vi "Add DataRow to Table by Values.vi"(8 "error in (no error)":errorcluster caption="错误输入（无错误）", 10 "values":variant[](array[variant]), 11 "DataTable 输入":refnum<class "DataTable.lvclass"> caption="DNL_LabVIEW Object in") -> (0 "error out":errorcluster caption="错误输出", 3 "DataTable 输出":refnum<class "DataTable.lvclass"> caption="DNL_LabVIEW Object out")   [LabVIEW 2012, in "Data Grid VIEW.lvlib" / "DataTable.lvclass"]
uses:
  DataTable.lvclass
  DataTable.lvclass/DataTable.ctl
  System.Data
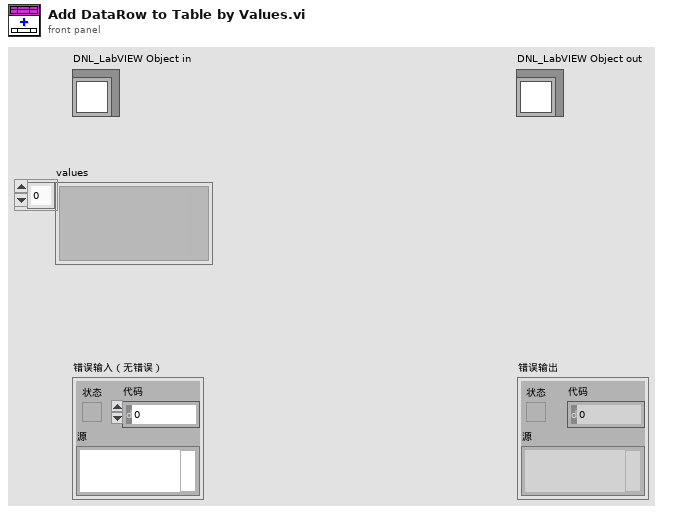
[diagram p1: front panel]
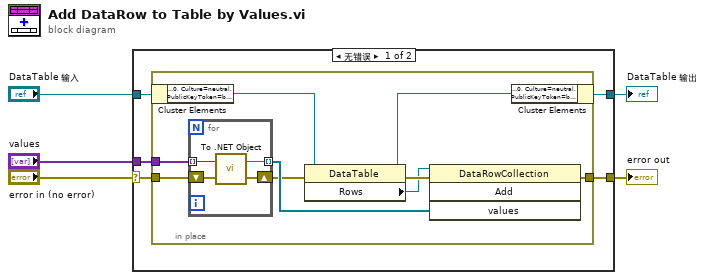
[diagram p0: block diagram]
diagram:
  n1 = case shown="无错误" "error in (no error)" {
    selector: "error in (no error)" -> [w8 w25]
    tunnel: [w7 w25] -> w4
    tunnel: [w6 w24] -> w2
    tunnel: "DataTable 输入" -> [w10 w24]
    tunnel: "values" -> [w9 _]
    frame No Error {
      n2 = in-place {
        in-place-border: w9 -> [w15]
        in-place-border: w8 -> [w13]
        in-place-border: [w11] -> w7
        n3 = in-place-cluster #1(w10) -> ("DataTable"=w17:refnum<k24>)
        n4 = for {
          tunnel: w15 -> [w23] mode=indexing
          tunnel: [w22] -> w14 mode=indexing
          shift-right: [w20] -> w12
          shift-left: w13 -> [w21]
          n5 = call <vilib>:"To .NET Object.vi"("error in (no error)"=w21, "anything"=w23) -> ("error out"=w20:errorcluster, ".NET object"=w22:refnum<k24>)
        }
        n6 = property class="DataTable"(reference=w17, error in=w12) -> (reference out=w16:refnum<k24>, error out=w19:errorcluster, "Rows"=w18:refnum<k24>)
        n7 = invoke class="DataRowCollection" method="Add"(reference=w18, error in=w19, "values"=w14) -> (error out=w11:errorcluster)  [unwired: 1 in, 3 out]
        n8 = in-place-cluster #1("DataTable"=w16) -> (w6:refnum<class "DataTable.lvclass">)
      }
    }
    frame Error {
    }
  }
  "error out" <- w4
  "DataTable 输出" <- w2
